vi "Save Log Config to Preferences.vi"(8 "error in (no error)":errorcluster, 11 "User Preferences File in":refnum<class "User Preferences File.lvclass">) -> (0 "error out":errorcluster, 3 "User Preferences File out":refnum<class "User Preferences File.lvclass">)   [LabVIEW 2020, in "RxnRover.lvlib"]
doc: "Stores the log configuration to the provided user preferences object. It does not save the user preferences to a file! This VI serves as a link between a User Preferences File object and the logging library without directly coupling the two.\n\nNOTE: The provided User Preferences object must already be initialized.\n\nTo view or update the log configuration at runtime, use the logging.lvlib:Set Log Config.vi and logging.lvlib:Get Log Config.vi VIs."
uses:
  RxnRover.lvlib
  User Preferences/User Preferences File.lvclass
  logging.lvlib
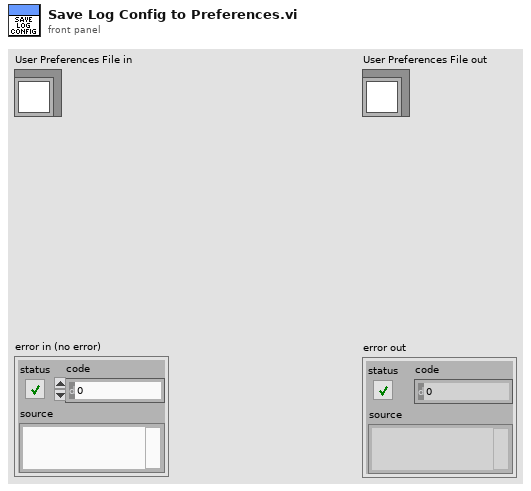
[diagram p1: front panel]
types:
  T1 = typedef "RxnRover.lvlib/logging.lvlib/Log Config.ctl" = cluster{"Log Level":T2}
  T2 = typedef "RxnRover.lvlib/logging.lvlib/Log Levels.ctl" = enum16{"NOTSET", "DEBUG", "INFO", "WARNING", "ERROR", "CRITICAL"}
  T3 = typedef "RxnRover.lvlib/User Preferences File.lvclass/User Preferences Cluster.ctl" = cluster{"Max Recent Experiments":dbl, "Recent Experiments":string[], "Log Level":string}
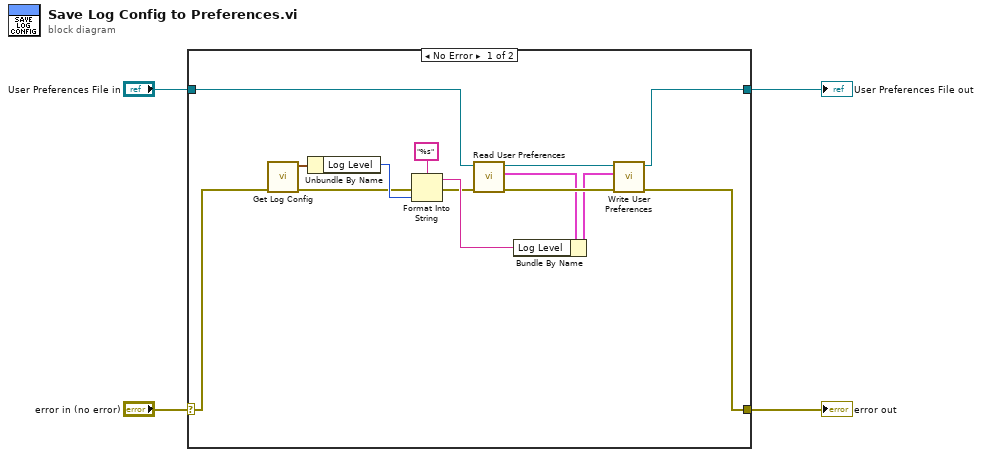
[diagram p0: block diagram]
diagram:
  n1 = case shown="No Error" "error in (no error)" {
    selector: "error in (no error)" -> [w18 w20]
    tunnel: [w5 w20] -> w4
    tunnel: "User Preferences File in" -> [w13 w19]
    tunnel: [w12 w19] -> w1
    frame No Error {
      n2 = call "Get Log Config.vi"("error in (no error)"=w18) -> ("error out"=w7:errorcluster, "Log Config"=w11:T1)  [unwired: 9 in]
      n3 = Unbundle By Name(w11) -> ("Log Level"=w10:T2)
      n4 = Format Into String(format string="%s", error in=w7, w10) -> (resulting string=w8:string, error out=w6:errorcluster)  [unwired: 1 in]
      n5 = call-dynamic "Read User Preferences.vi"("error in (no error)"=w6, "User Preferences File in"=w13) -> ("error out"=w17:errorcluster, "User Preferences"=w16:T3, "User Preferences File out"=w14:refnum<class "User Preferences File.lvclass">)  [unwired: 7 in]
      n6 = Bundle By Name(cluster=w16, "Log Level"=w8) -> (w15:T3)
      n7 = call-dynamic "Write User Preferences.vi"("error in (no error)"=w17, "User Preferences"=w15, "User Preferences File in"=w14) -> ("error out"=w5:errorcluster, "User Preferences File out"=w12:refnum<class "User Preferences File.lvclass">)  [unwired: 7 in]
    }
    frame Error {
    }
  }
  "error out" <- w4
  "User Preferences File out" <- w1
